vi "ActionVIOnLoad.vi"(8 "error in (no error)":errorcluster, 11 "Device Item Ref in":T1 format="%.0x") -> (0 "error out":errorcluster, 3 "Device Item Ref out":T1 format="%.0x")   [LabVIEW 2015, in "Diagnostics Addon System Explorer.lvlib"]
uses:
  Diagnostics Addon System Explorer.lvlib
  <vilib>/NI Veristand/Custom Device API/Custom Device Item Ref.ctl
  Shared/Types/Signal.ctl
  Shared/Types/986x.ctl
  Types/FG.Action.ctl
  Shared/Types/CAN.ctl
  Shared/Types/CAN.Interface.ctl
  Shared/Types/Protocol.ctl
  Shared/Types/Transport.ctl
  Shared/Types/Security.ctl
  Shared/Types/Type.ctl
  <vilib>/NI Veristand/Custom Device API/Custom Device Channel.ctl
  <vilib>/NI Veristand/Custom Device API/Custom Device Channel Type.ctl
  NationalInstruments.VeriStand.SystemDefinitionAPI
  SubVIs/FileDependency.Create.vi
  SubVIs/ID.FG.vi
  Shared/SubVIs/Constants.vi
  <vilib>/NI Veristand/Custom Device Tools/Custom Device Utility Library/NI VeriStand - Search for All Items by GUID.vi
  <vilib>/NI Veristand/Custom Device API/Get Item Property (Variant).vi
  <vilib>/NI Veristand/Custom Device API/Set Item Property (Variant).vi
  <vilib>/NI Veristand/Custom Device API/Get Item Property (U32).vi
  <vilib>/NI Veristand/Custom Device API/Get Item Property (Boolean).vi
  SubVIs/FileDependency.Get.Target Path.vi
  <vilib>/NI/NIVS System Definition Utilities/SysDef API/SysDef.Property.Set.vi
  <vilib>/NI/NIVS System Definition Utilities/_SubVIs/SysDef.Property.Set.U32.vi
  <vilib>/NI/NIVS System Definition Utilities/_SubVIs/SysDef.Property.Set.Boolean.vi
  <vilib>/Utility/MD5Checksum.llb/MD5Checksum File.vi
  <vilib>/NI/NIVS System Definition Utilities/_SubVIs/SysDef.Property.Set.DependentFile.vi
  <vilib>/NI/NIVS System Definition Utilities/SysDef API/SysDef.Property.Remove.vi
  <vilib>/NI Veristand/Custom Device API/Get Item Property (U16).vi
  <vilib>/NI Veristand/Custom Device API/Get Item Property (Path).vi
  <vilib>/NI Veristand/Custom Device Tools/Custom Device Utility Library/NI VeriStand - Search for Item by GUID.vi
  <vilib>/NI/NIVS System Definition Utilities/_SubVIs/SysDef.Property.Set.I32.vi
  <vilib>/NI Veristand/Custom Device API/Get Item Property (I32).vi
  <vilib>/NI/NIVS System Definition Utilities/_SubVIs/SysDef.Property.Set.U32.Array.vi
  <vilib>/NI Veristand/Custom Device API/Get Item Property (U32 Array).vi
  Shared/Diagnostics Addon Shared.lvlib
  <vilib>/NI VeriStand/Custom Device API/Custom Device API.lvlib
  <vilib>/NI Veristand/Custom Device Tools/Custom Device Utility Library/Custom Device Utility Library.lvlib
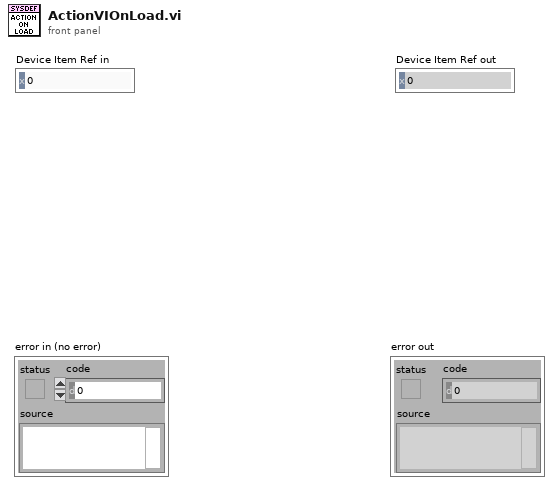
[diagram p1: front panel]
types:
  T1 = typedef "Custom Device API.lvlib/Custom Device Item Ref.ctl" = u64
  T2 = typedef "Diagnostics Addon Shared.lvlib/Signal.ctl" = cluster{"Start Bit":u32, "Length":u32, "Scaling Factor":dbl, "Scaling Offset":dbl, "Minimum":dbl, "Maximum":dbl, "Data Type":u32, "Byte Order":u32, "Default Value":dbl, "Name":string, "Units":string, "Description":string}
  T3 = cluster{"Name":string, "Start Bit":u8, "Length":u8, "Scaling Factor":dbl, "Scaling Offset":dbl, "Minimum":dbl, "Maximum":dbl, "Data Type":u32, "Byte Order":u32, "Default Value":dbl, "Units":string, "Description":string}
  T4 = cluster{"Start Bit":u8, "Length":u8, "Scaling Factor":dbl, "Scaling Offset":dbl, "Minimum":dbl, "Maximum":dbl, "Data Type":u32, "Byte Order":u32, "Default Value":dbl, "Name":string, "Units":string, "Description":string}
  T5 = typedef "Diagnostics Addon System Explorer.lvlib/FG.Action.ctl" = enum16{"Get", "Set"}
  T6 = typedef "Diagnostics Addon Shared.lvlib/986x.ctl" = cluster{"Enable":bool, "RIO Device":u16, "Bitfile":path}
  T7 = typedef "Custom Device API.lvlib/Custom Device Channel.ctl" = cluster{"Type":T8, "Units":string, "Default Value":dbl, "Faultable":bool, "Scalable":bool}
  T8 = typedef "Custom Device API.lvlib/Custom Device Channel Type.ctl" = enum16{"Input", "Output"}
  T9 = typedef "Diagnostics Addon Shared.lvlib/Type.ctl" = enum16{"DID", "CDID", "PID", "CPID", "Read Memory", "Write Memory", "DTC Control", "IO Cmd", "IO Resp", "Routine Start Cmd", "Routine Start Resp", "Routine Request Cmd", "Routine Request Resp", "Routine Stop Cmd", "Routine Stop Resp", "UserDefined Cmd", "UserDefined Rsp"}
  T10 = typedef "Diagnostics Addon Shared.lvlib/CAN.ctl" = cluster{"CAN Interface":T11, "Baud Rate":u32, "Diagnostic Protocol":T12, "Transport Protocol":T13, "Transmit ID":u32, "Receive ID":u32, "Transmit Extension":u8, "Receive Extension":u8, "Receive UUDT ID":u32, "Enable Stream":bool, "VW TP Channel ID":u32, "Security":T14, "Fill Frame":bool, "Fill Byte":u8, "Termination":bool}
  T11 = typedef "Diagnostics Addon Shared.lvlib/CAN.Interface.ctl" = enum16{"CAN0", "CAN1", "CAN2", "CAN3", "CAN4", "CAN5", "CAN6", "CAN7", "CAN8", "CAN9", "CAN10", "CAN11", "CAN12", "CAN13", "CAN14", "CAN15", "CAN16", "CAN17", "CAN18", "CAN19", "CAN20", "CAN21", "CAN22", "CAN23", "CAN24", "CAN25", "CAN26", "CAN27", "CAN28", "CAN29", "CAN30", "CAN31", "CAN32", "CAN33", "CAN34", "CAN35", "CAN36", "CAN37", "CAN38", "CAN39", "CAN40", "CAN41", "CAN42", "CAN43", "CAN44", "CAN45", "CAN46", "CAN47", "CAN48", "CAN49", "CAN50", "CAN51", "CAN52", "CAN53", "CAN54", "CAN55", "CAN56", "CAN57", "CAN58", "CAN59", "CAN60", "CAN61", "CAN62", "CAN63", "CAN 256 (Virtual)", "CAN 257 (Virtual)"}
  T12 = typedef "Diagnostics Addon Shared.lvlib/Protocol.ctl" = enum16{"GMLAN", "KWP-2000", "UDS", "User-Defined"}
  T13 = typedef "Diagnostics Addon Shared.lvlib/Transport.ctl" = enum16{"ISO TP - Normal Mode", "ISO TP - Mixed Mode", "VW TP 2.0", "Diagnostics on IP"}
  T14 = typedef "Diagnostics Addon Shared.lvlib/Security.ctl" = cluster{"Source DLL Path":path, "Security Level":u8, "Target DLL Path":path}
  T15 = cluster{"DTC Byte Length":i32, "Status Byte Length":i32, "Add Data Byte Length":i32, "Byte Order":enum16{"Motorola", "Intel"}}
  T16 = cluster{"Database File":path, "CAN Interface":enum16{"CAN0", "CAN1", "CAN2", "CAN3", "CAN4", "CAN5", "CAN6", "CAN7", "CAN8", "CAN9", "CAN10", "CAN11", "CAN12", "CAN13", "CAN14", "CAN15", "CAN16", "CAN17", "CAN18", "CAN19", "CAN20", "CAN21", "CAN22", "CAN23", "CAN24", "CAN25", "CAN26", "CAN27", "CAN28", "CAN29", "CAN30", "CAN31", "CAN32", "CAN33", "CAN34", "CAN35", "CAN36", "CAN37", "CAN38", "CAN39", "CAN40", "CAN41", "CAN42", "CAN43", "CAN44", "CAN45", "CAN46", "CAN47", "CAN48", "CAN49", "CAN50", "CAN51", "CAN52", "CAN53", "CAN54", "CAN55", "CAN56", "CAN57", "CAN58", "CAN59", "CAN60", "CAN61", "CAN62", "CAN63", "CAN 256 (Virtual)", "CAN 257 (Virtual)"}, "Baud Rate":u32, "Diagnostic Protocol":enum16{"GMLAN", "KWP-2000", "UDS"}, "Transport Protocol":enum16{"ISO TP - Normal Mode", "ISO TP - Mixed Mode", "VW TP 2.0", "Diagnostics on IP"}, "Transmit ID":u32, "Receive ID":u32, "Transmit Extension":u8, "Receive Extension":u8, "Receive UUDT ID":u32, "Enable Stream":bool, "VW TP Channel ID":u32}
  T17 = enum16{"CAN0", "CAN1", "CAN2", "CAN3", "CAN4", "CAN5", "CAN6", "CAN7", "CAN8", "CAN9", "CAN10", "CAN11", "CAN12", "CAN13", "CAN14", "CAN15", "CAN16", "CAN17", "CAN18", "CAN19", "CAN20", "CAN21", "CAN22", "CAN23", "CAN24", "CAN25", "CAN26", "CAN27", "CAN28", "CAN29", "CAN30", "CAN31", "CAN32", "CAN33", "CAN34", "CAN35", "CAN36", "CAN37", "CAN38", "CAN39", "CAN40", "CAN41", "CAN42", "CAN43", "CAN44", "CAN45", "CAN46", "CAN47", "CAN48", "CAN49", "CAN50", "CAN51", "CAN52", "CAN53", "CAN54", "CAN55", "CAN56", "CAN57", "CAN58", "CAN59", "CAN60", "CAN61", "CAN62", "CAN63", "CAN 256 (Virtual)", "CAN 257 (Virtual)"}
  T18 = enum16{"ISO TP - Normal Mode", "ISO TP - Mixed Mode", "VW TP 2.0", "Diagnostics on IP"}
  T19 = cluster{"DPID ID":u8, "Speed":enum16{"Slow", "Medium", "Fast"}, "PIDs":u16[]}
  T20 = typedef "Custom Device API.lvlib/Custom Device Item Info.ctl" = cluster{"Name":string, "Is Channel":bool, "GUID":string, "Is Waveform":bool}
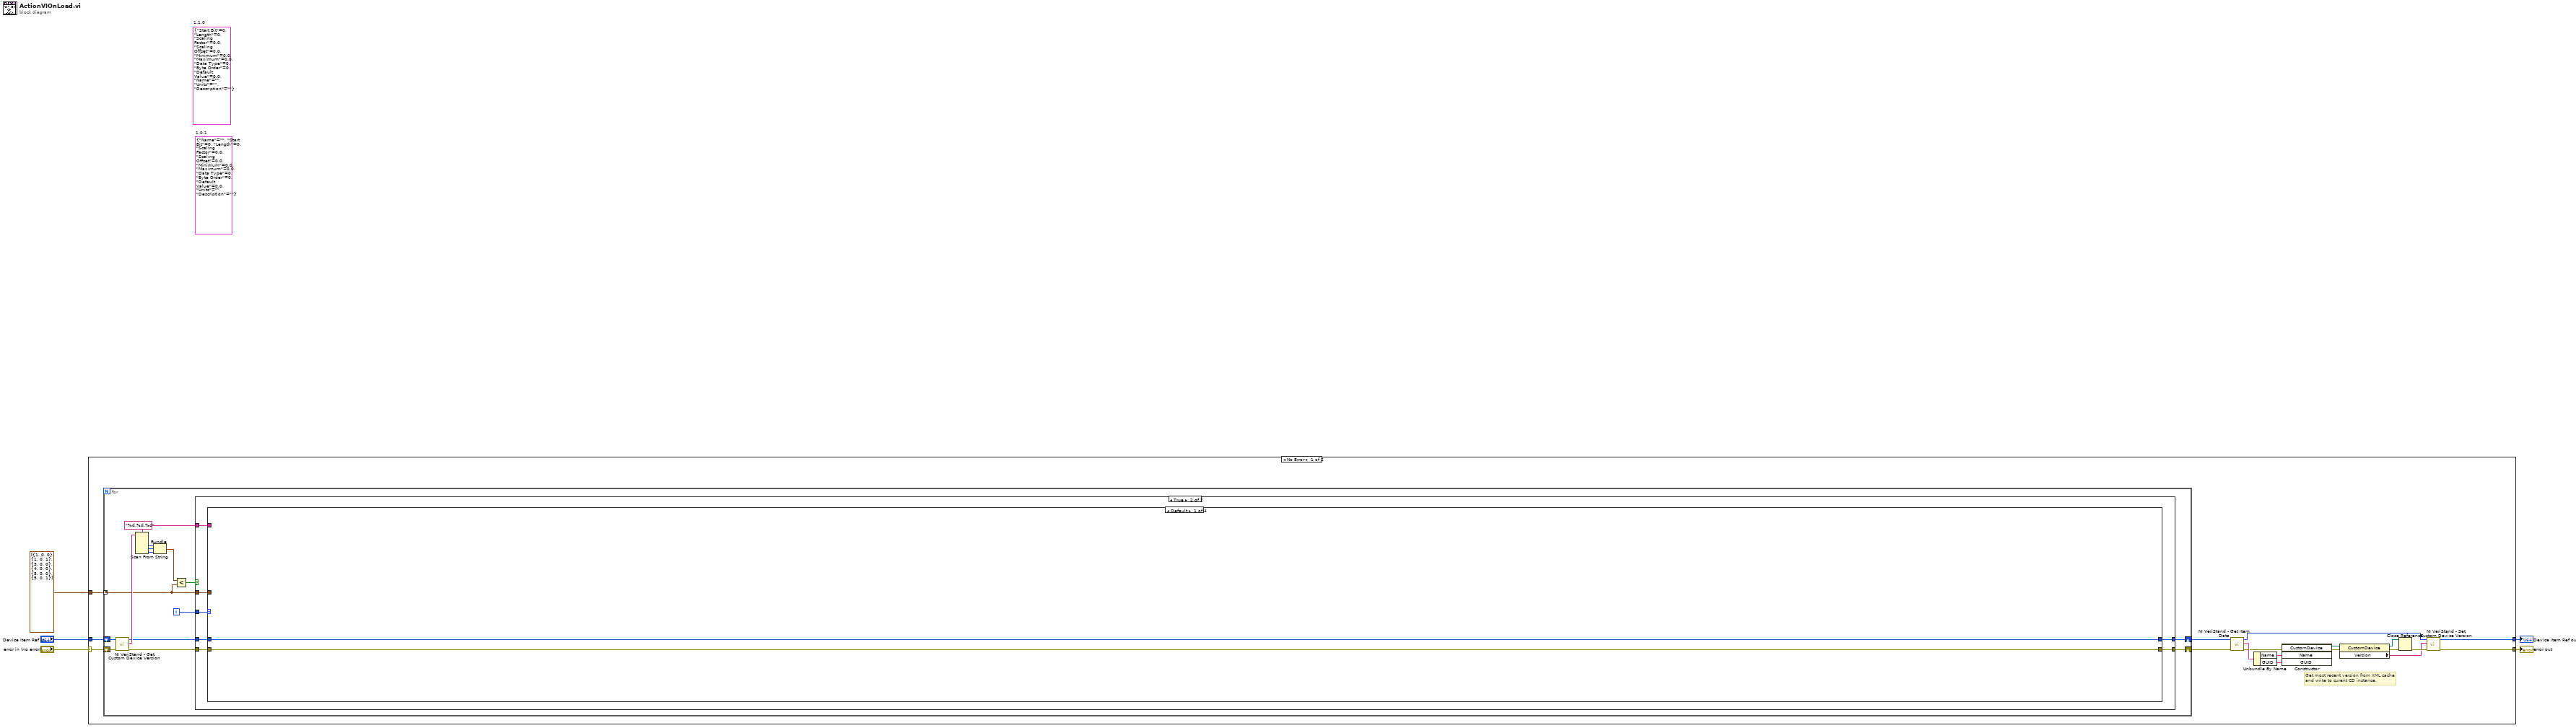
[diagram p0: block diagram]
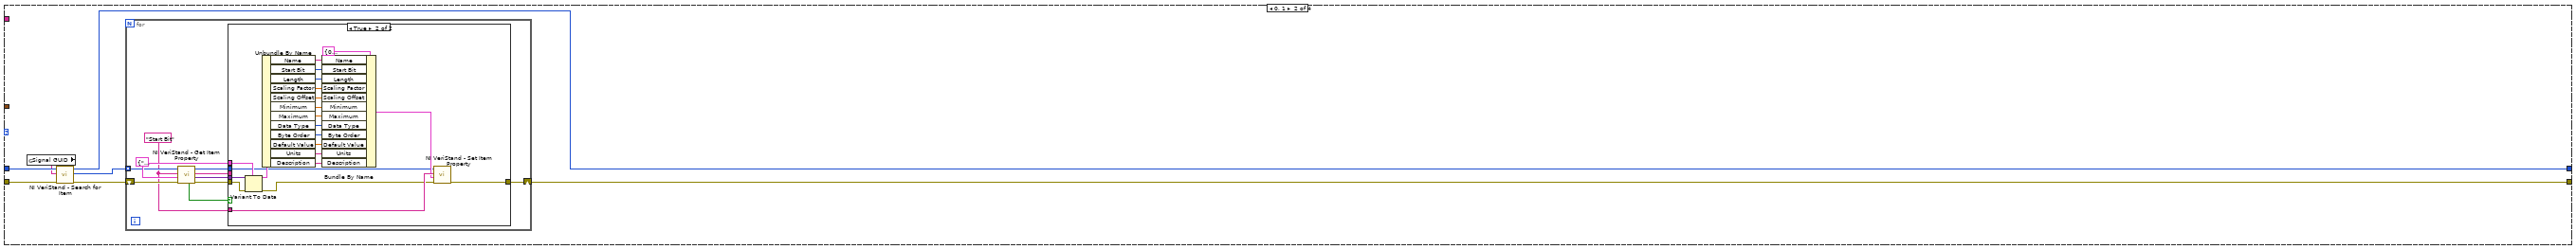
[diagram p3: hidden frame]
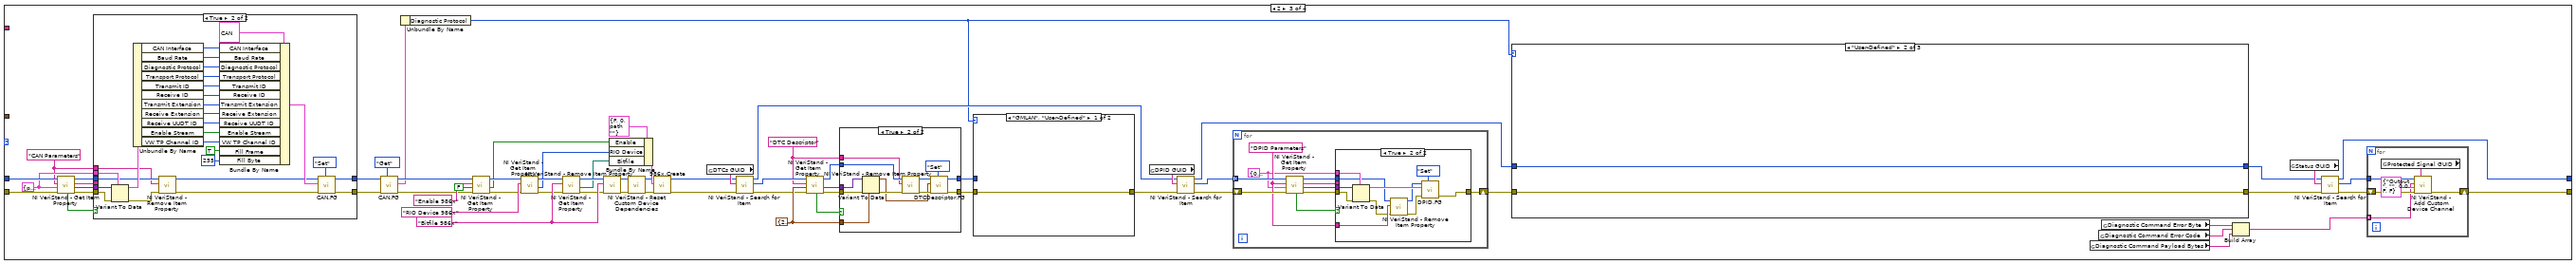
[diagram p5: hidden frame]
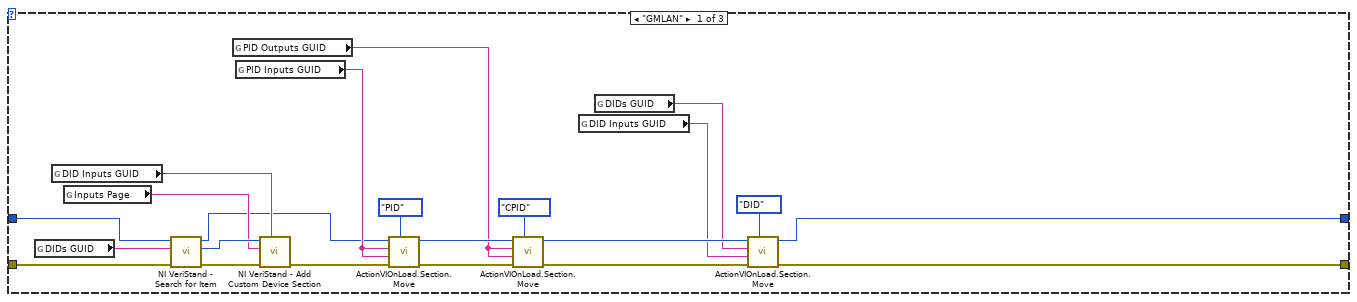
[diagram p6: hidden frame]
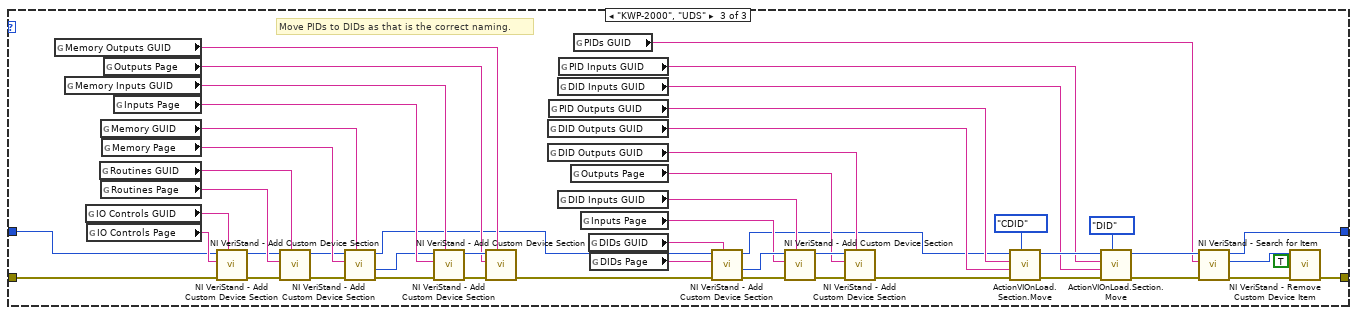
[diagram p7: hidden frame]
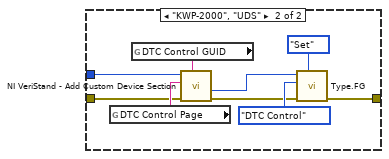
[diagram p8: hidden frame]
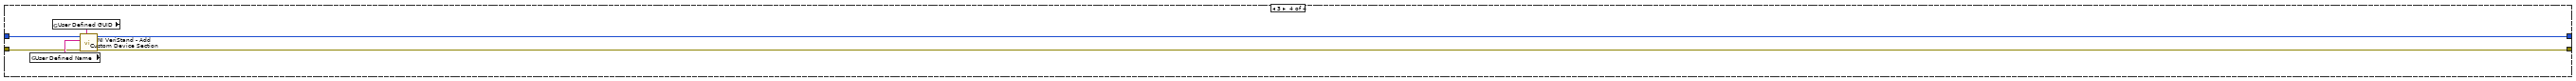
[diagram p12: hidden frame]
diagram:
  (unwired) T2 {"Start Bit"=0, "Length"=0, "Scaling Factor"=0.0, "Scaling Offset"=0.0, "Minimum"=0.0, "Maximum"=0.0, "Data Type"=0, "Byte Order"=0, "Default Value"=0.0, "Name"="", "Units"="", "Description"=""}  # 1.1.0
  (unwired) T3 {"Name"="", "Start Bit"=0, "Length"=0, "Scaling Factor"=0.0, "Scaling Offset"=0.0, "Minimum"=0.0, "Maximum"=0.0, "Data Type"=0, "Byte Order"=0, "Default Value"=0.0, "Units"="", "Description"=""}  # 1.0.1
  n1 = case shown="No Error" "error in (no error)" {
    selector: "error in (no error)" -> [w22 w315]
    tunnel: [w8 w315] -> w2
    tunnel: "Device Item Ref in" -> [w21 w314]
    tunnel: [w6 w314] -> w1
    tunnel: cluster{i32, i32, i32}[] [{1, 0, 0}, {1, 0, 1}, {3, 0, 0}, {4, 0, 0}, {5, 0, 0}, {5, 0, 1}] -> [w23 _]
    frame No Error {
      # "Get most recent version from XML cache\nand write to curent CD instance."
      n2 = for {
        tunnel: w23 -> [w26] mode=indexing
        shift-right: [w31] -> w9
        shift-left: w22 -> [w36]
        shift-right: [w29] -> w7
        shift-left: w21 -> [w35]
        i -> [w28]
        w27 = "%d.%d.%d" ("format string")
        n3 = call <vilib>:"NI VeriStand - Get Custom Device Version.vi"("error in (no error)"=w36, "Device Ref in"=w35) -> ("error out"=w32:errorcluster, "Value"=w34:string, "Device Ref out"=w30:T1)  [unwired: 7 in]
        n4 = Scan From String(format string=w27, input string=w34) -> (output 1=w37:i32, output 2=w38:i32, output 3=w25:i32)  [unwired: 5 in, 3 out]
        n5 = Bundle(w37, w38, w25) -> (w24:cluster{i32, i32, i32})  [unwired: 1 in]
        n6 = Less?(x=w24, y=w26) -> (x < y?=w33:bool)
        n7 = case shown="True" w33 {
          tunnel: w32 -> [w40 w47]
          tunnel: [w40 w46] -> w31
          tunnel: w30 -> [w39 w43]
          tunnel: [w39 w44] -> w29
          tunnel: w28 -> [_ w45]
          tunnel: w26 -> [_ w42]
          tunnel: w27 -> [_ w41]
          frame False {
          }
          frame True {
            n8 = case shown="Default" w45 {
              tunnel: w47 -> [w49 w55 w149 w311]
              tunnel: [w49 w51 w90 w309] -> w46
              tunnel: [w48 w50 w89 w308] -> w44
              tunnel: w43 -> [w48 w56 w148 w310]
              tunnel: w42 -> [_ _ _ _]
              tunnel: w41 -> [_ _ _ _]
              frame Default {
              }
              frame 0, 1 {
                n9 = global read "Constants.vi" "Signal GUID"() -> (w54:string)
                n10 = call-poly <vilib>:"NI VeriStand - Search for Item.vi"("error in"=w55, "Item GUID"=w54, "Section Ref in"=w56) -> ("error out"=w53:errorcluster, "Item Refs"=w52:T1[], "Section Ref out"=w50:T1)  [unwired: 5 in, 1 out]
                n11 = for {
                  shift-right: [w60] -> w51
                  shift-left: w53 -> [w61]
                  tunnel: w52 -> [w58] mode=indexing
                  w57 = "Start Bit" ("DIDPID Signal Parameters")
                  w62 = T3 {"Name"="", "Start Bit"=0, "Length"=0, "Scaling Factor"=0.0, "Scaling Offset"=0.0, "Minimum"=0.0, "Maximum"=0.0, "Data Type"=0, "Byte Order"=0, "Default Value"=0.0, "Units"="", "Description"=""} ("Signal Parameters")
                  n12 = call-poly <vilib>:"NI VeriStand - Get Item Property.vi"("error in (no error)"=w61, "Default Value"=w62, "Property Name"=w57, "Item Ref in"=w58) -> ("error out"=w64:errorcluster, "Value"=w63:variant, "Item Ref out"=w59:T1, "Found?"=w65:bool)  [unwired: 4 in]
                  n13 = case shown="True" w65 {
                    tunnel: w64 -> [w66 w88]
                    tunnel: w63 -> [_ w87]
                    tunnel: w62 -> [_ w86]
                    tunnel: [w66 w67] -> w60
                    tunnel: w59 -> [_ w69]
                    tunnel: w57 -> [_ _]
                    tunnel: w57 -> [_ w71]
                    frame False {
                    }
                    frame True {
                      n14 = Variant To Data(error in=w88, type=w86, Variant=w87) -> (data=w85:T3, error out=w68:errorcluster)
                      n15 = Unbundle By Name(w85) -> ("Name"=w84:string, "Start Bit"=w83:u8, "Length"=w82:u8, "Scaling Factor"=w81:dbl, "Scaling Offset"=w80:dbl, "Minimum"=w79:dbl, "Maximum"=w78:dbl, "Data Type"=w77:u32, "Byte Order"=w76:u32, "Default Value"=w75:dbl, "Units"=w74:string, "Description"=w73:string)
                      n16 = Bundle By Name(cluster=T4 {"Start Bit"=0, "Length"=0, "Scaling Factor"=0.0, "Scaling Offset"=0.0, "Minimum"=0.0, "Maximum"=0.0, "Data Type"=0, "Byte Order"=0, "Default Value"=0.0, "Name"="", "Units"="", "Description"=""} ("Signal Parameters"), "Name"=w84, "Start Bit"=w83, "Length"=w82, "Scaling Factor"=w81, "Scaling Offset"=w80, "Minimum"=w79, "Maximum"=w78, "Data Type"=w77, "Byte Order"=w76, "Default Value"=w75, "Units"=w74, "Description"=w73) -> (w70:T4)
                      n17 = call-poly <vilib>:"NI VeriStand - Set Item Property.vi"("error in (no error)"=w68, "Value"=w70, "Property Name"=w71, "Item Ref in"=w69) -> ("error out"=w67:errorcluster)  [unwired: 5 in, 2 out]
                    }
                  }
                }
              }
              frame 2 {
                w129 = T15 {"DTC Byte Length"=2, "Status Byte Length"=1, "Add Data Byte Length"=1, "Byte Order"=enum."Motorola"} ("DTC descriptor")
                w122 = "DTC Descriptor" ("DTC Descriptor")
                w143 = "Bitfile 986x" ("Bitfile 986x")
                w106 = "CAN Parameters" ("DIDPID Signal Parameters")
                w147 = T16 {"Database File"=path "", "CAN Interface"=enum."CAN0", "Baud Rate"=0, "Diagnostic Protocol"=enum."GMLAN", "Transport Protocol"=enum."ISO TP - Normal Mode", "Transmit ID"=0, "Receive ID"=0, "Transmit Extension"=0, "Receive Extension"=0, "Receive UUDT ID"=0, "Enable Stream"=TRUE, "VW TP Channel ID"=0} ("Diagnostics Basic Configuraiton")
                n18 = call-poly <vilib>:"NI VeriStand - Get Item Property.vi"("error in (no error)"=w149, "Default Value"=w147, "Property Name"=w106, "Item Ref in"=w148) -> ("error out"=w152:errorcluster, "Value"=w151:variant, "Item Ref out"=w150:T1, "Found?"=w153:bool)  [unwired: 4 in]
                n19 = case shown="True" w153 {
                  tunnel: w152 -> [w280 w307]
                  tunnel: w151 -> [_ w306]
                  tunnel: w147 -> [_ w305]
                  tunnel: [w280 w290] -> w112
                  tunnel: w150 -> [w279 w283]
                  tunnel: w106 -> [_ _]
                  tunnel: [w279 w288] -> w110
                  tunnel: w106 -> [_ w281]
                  frame False {
                  }
                  frame True {
                    n20 = Variant To Data(error in=w307, type=w305, Variant=w306) -> (data=w304:T16, error out=w285:errorcluster)
                    n21 = Unbundle By Name(w304) -> ("CAN Interface"=w303:T17, "Baud Rate"=w302:u32, "Diagnostic Protocol"=w301:enum16{"GMLAN", "KWP-2000", "UDS"}, "Transport Protocol"=w300:T18, "Transmit ID"=w299:u32, "Receive ID"=w298:u32, "Transmit Extension"=w297:u8, "Receive Extension"=w296:u8, "Receive UUDT ID"=w295:u32, "Enable Stream"=w294:bool, "VW TP Channel ID"=w293:u32)
                    n22 = call <vilib>:"NI VeriStand - Remove Item Property.vi"("error in (no error)"=w285, "Property Name"=w281, "Item Ref in"=w283) -> ("error out"=w284:errorcluster, "Item Ref out"=w282:T1)  [unwired: 6 in, 1 out]
                    n23 = Bundle By Name(cluster=T10 {"CAN Interface"=enum."CAN0", "Baud Rate"=0, "Diagnostic Protocol"=enum."GMLAN", "Transport Protocol"=enum."ISO TP - Normal Mode", "Transmit ID"=0, "Receive ID"=0, "Transmit Extension"=0, "Receive Extension"=0, "Receive UUDT ID"=0, "Enable Stream"=TRUE, "VW TP Channel ID"=0, "Security"={"Source DLL Path"=path "", "Security Level"=1, "Target DLL Path"=path ""}, "Fill Frame"=FALSE, "Fill Byte"=255, "Termination"=FALSE} ("Diagnostics Basic Configuraiton"), "CAN Interface"=w303, "Baud Rate"=w302, "Diagnostic Protocol"=w301, "Transport Protocol"=w300, "Transmit ID"=w299, "Receive ID"=w298, "Transmit Extension"=w297, "Receive Extension"=w296, "Receive UUDT ID"=w295, "Enable Stream"=w294, "VW TP Channel ID"=w293, "Fill Frame"=TRUE, "Fill Byte"=u8 255) -> (w289:T10)
                    n24 = call "CAN.FG.vi"("Action"=FG.Action."Set", "error in (no error)"=w284, "Diagnostics Basic Configuraiton"=w289, "Device Item Ref in"=w282) -> ("error out"=w290:errorcluster, "Device Item Ref out"=w288:T1)  [unwired: 5 in, 1 out]
                  }
                }
                n25 = call "CAN.FG.vi"("Action"=FG.Action."Get", "error in (no error)"=w112, "Device Item Ref in"=w110) -> ("error out"=w111:errorcluster, "Diagnostics Basic Configuraiton"=w108:T10, "Device Item Ref out"=w109:T1)  [unwired: 6 in]
                n26 = Unbundle By Name(w108) -> ("Diagnostic Protocol"=w91:T12)
                n27 = call-poly <vilib>:"NI VeriStand - Get Item Property.vi"("error in (no error)"=w111, "Default Value"=FALSE, "Property Name"="Enable 986x" ("Enable 986x"), "Item Ref in"=w109) -> ("error out"=w140:errorcluster, "Value"=w136:bool, "Item Ref out"=w139:T1)  [unwired: 4 in, 1 out]
                n28 = call-poly <vilib>:"NI VeriStand - Get Item Property.vi"("error in (no error)"=w140, "Property Name"="RIO Device 986x" ("RIO Device 986x"), "Item Ref in"=w139) -> ("error out"=w141:errorcluster, "Value"=w135:u16, "Item Ref out"=w138:T1)  [unwired: 5 in, 1 out]
                n29 = call-poly <vilib>:"NI VeriStand - Get Item Property.vi"("error in (no error)"=w141, "Property Name"=w143, "Item Ref in"=w138) -> ("error out"=w142:errorcluster, "Value"=w134:path, "Item Ref out"=w144:T1)  [unwired: 5 in, 1 out]
                n30 = call <vilib>:"NI VeriStand - Remove Item Property.vi"("error in (no error)"=w142, "Property Name"=w143, "Item Ref in"=w144) -> ("error out"=w102:errorcluster, "Item Ref out"=w132:T1)  [unwired: 6 in, 1 out]
                n31 = Bundle By Name(cluster=T6 {"Enable"=FALSE, "RIO Device"=0, "Bitfile"=path ""} ("986x Support"), "Enable"=w136, "RIO Device"=w135, "Bitfile"=w134) -> (w133:T6)
                n32 = call <vilib>:"NI VeriStand - Reset Custom Device Dependencies.vi"("error in (no error)"=w102, "Device Ref in"=w132) -> ("error out"=w101:errorcluster, "Device Ref out"=w103:T1)  [unwired: 8 in]
                n33 = call "986x.Create.vi"("error in (no error)"=w101, "986x Support"=w133, "Device Item Ref in"=w103) -> ("error out"=w105:errorcluster, "Device Ref out"=w104:T1)  [unwired: 7 in]
                n34 = global read "Constants.vi" "DTCs GUID"() -> (w130:string)
                n35 = call-poly <vilib>:"NI VeriStand - Search for Item.vi"("error in"=w105, "Item GUID"=w130, "Section Ref in"=w104) -> ("error out"=w125:errorcluster, "Item Ref"=w124:T1, "Section Ref out"=w115:T1)  [unwired: 5 in, 1 out]
                n36 = call-poly <vilib>:"NI VeriStand - Get Item Property.vi"("error in (no error)"=w125, "Default Value"=w129, "Property Name"=w122, "Item Ref in"=w124) -> ("error out"=w128:errorcluster, "Value"=w127:variant, "Item Ref out"=w123:T1, "Found?"=w126:bool)  [unwired: 4 in]
                n37 = case shown="True" w126 {
                  tunnel: w128 -> [w266 w278]
                  tunnel: [w266 w269] -> w118
                  tunnel: w127 -> [_ w277]
                  tunnel: w129 -> [_ w276]
                  tunnel: w123 -> [w265 w274]
                  tunnel: w122 -> [_ w268]
                  tunnel: [w265 w267] -> w117
                  frame False {
                  }
                  frame True {
                    n38 = Variant To Data(error in=w278, type=w276, Variant=w277) -> (data=w270:T15, error out=w275:errorcluster)
                    n39 = call <vilib>:"NI VeriStand - Remove Item Property.vi"("error in (no error)"=w275, "Property Name"=w268, "Item Ref in"=w274) -> ("error out"=w271:errorcluster, "Item Ref out"=w272:T1)  [unwired: 6 in, 1 out]
                    n40 = call "DTCDescriptor.FG.vi"("Action"=FG.Action."Set", "error in (no error)"=w271, "DTC descriptor"=w270, "Device Item Ref in"=w272) -> ("error out"=w269:errorcluster, "Device Item Ref out"=w267:T1)  [unwired: 5 in, 1 out]
                  }
                }
                n41 = case shown="\"GMLAN\", \"User-Defined\"" w91 {
                  tunnel: w118 -> [w234 w238]
                  tunnel: w117 -> [_ w237]
                  tunnel: [w234 w236] -> w116
                  frame "GMLAN", "User-Defined" {
                  }
                  frame "KWP-2000", "UDS" {
                    n42 = global read "Constants.vi" "DTC Control Page"() -> (w243:string)
                    n43 = global read "Constants.vi" "DTC Control GUID"() -> (w242:string)
                    n44 = call <vilib>:"NI VeriStand - Add Custom Device Section.vi"("GUID (Default Section)"=w242, "error in (no error)"=w238, "Section Name"=w243, "Parent Ref in"=w237) -> ("error out"=w239:errorcluster, "Section Ptr"=w235:T1)  [unwired: 4 in, 2 out]
                    n45 = call "Type.FG.vi"("Action"=FG.Action."Set", "error in (no error)"=w239, "Type"=Type."DTC Control", "Device Item Ref in"=w235) -> ("error out"=w236:errorcluster)  [unwired: 5 in, 2 out]
                  }
                }
                n46 = global read "Constants.vi" "DPID GUID"() -> (w120:string)
                n47 = call-poly <vilib>:"NI VeriStand - Search for Item.vi"("error in"=w116, "Item GUID"=w120, "Section Ref in"=w115) -> ("error out"=w119:errorcluster, "Item Refs"=w121:T1[], "Section Ref out"=w107:T1)  [unwired: 5 in, 1 out]
                n48 = for {
                  shift-right: [w248] -> w114
                  shift-left: w119 -> [w249]
                  tunnel: w121 -> [w246] mode=indexing
                  w244 = T19 {"DPID ID"=0, "Speed"=enum."Slow", "PIDs"=[]} ("DPID")
                  w245 = "DPID Parameters" ("DPID Parameters")
                  n49 = call-poly <vilib>:"NI VeriStand - Get Item Property.vi"("error in (no error)"=w249, "Default Value"=w244, "Property Name"=w245, "Item Ref in"=w246) -> ("error out"=w251:errorcluster, "Value"=w250:variant, "Item Ref out"=w247:T1, "Found?"=w252:bool)  [unwired: 4 in]
                  n50 = case shown="True" w252 {
                    tunnel: w251 -> [w253 w264]
                    tunnel: w250 -> [_ w263]
                    tunnel: w244 -> [_ w262]
                    tunnel: [w253 w256] -> w248
                    tunnel: w247 -> [_ w255]
                    tunnel: w245 -> [_ _]
                    tunnel: w245 -> [_ w261]
                    frame False {
                    }
                    frame True {
                      n51 = Variant To Data(error in=w264, type=w262, Variant=w263) -> (data=w260:T19, error out=w258:errorcluster)
                      n52 = call <vilib>:"NI VeriStand - Remove Item Property.vi"("error in (no error)"=w258, "Property Name"=w261, "Item Ref in"=w255) -> ("error out"=w257:errorcluster, "Item Ref out"=w254:T1)  [unwired: 6 in, 1 out]
                      n53 = call "DPID.FG.vi"("Action"=FG.Action."Set", "error in (no error)"=w257, "DPID"=w260, "Device Item Ref in"=w254) -> ("error out"=w256:errorcluster)  [unwired: 5 in, 2 out]
                    }
                  }
                }
                n54 = case shown="\"User-Defined\"" w91 {
                  tunnel: [w168 w182 w189] -> w92
                  tunnel: [w164 w183 w185] -> w94
                  tunnel: w114 -> [w166 w183 w215]
                  tunnel: w107 -> [w180 w182 w214]
                  frame "GMLAN" {
                    n55 = global read "Constants.vi" "DIDs GUID"() -> (w181:string)
                    n56 = global read "Constants.vi" "DID Inputs GUID"() -> (w177:string)
                    n57 = global read "Constants.vi" "Inputs Page"() -> (w176:string)
                    n58 = call-poly <vilib>:"NI VeriStand - Search for Item.vi"("error in"=w166, "Item GUID"=w181, "Section Ref in"=w180) -> ("error out"=w179:errorcluster, "Item Ref"=w178:T1, "Section Ref out"=w163:T1)  [unwired: 5 in, 1 out]
                    n59 = global read "Constants.vi" "PID Outputs GUID"() -> (w170:string)
                    n60 = global read "Constants.vi" "PID Inputs GUID"() -> (w171:string)
                    n61 = call <vilib>:"NI VeriStand - Add Custom Device Section.vi"("GUID (Default Section)"=w177, "error in (no error)"=w179, "Section Name"=w176, "Parent Ref in"=w178) -> ("error out"=w165:errorcluster)  [unwired: 4 in, 3 out]
                    n62 = call "ActionVIOnLoad.Section.Move.vi"("Type"=Type."PID", "error in (no error)"=w165, "Paste Parent GUID"=w171, "Copy Parent GUID"=w171, "Section Ref in"=w163) -> ("error out"=w175:errorcluster, "Section Ref out"=w174:T1)  [unwired: 5 in]
                    n63 = call "ActionVIOnLoad.Section.Move.vi"("Type"=Type."CPID", "error in (no error)"=w175, "Paste Parent GUID"=w170, "Copy Parent GUID"=w170, "Section Ref in"=w174) -> ("error out"=w167:errorcluster, "Section Ref out"=w169:T1)  [unwired: 5 in]
                    n64 = global read "Constants.vi" "DID Inputs GUID"() -> (w161:string)
                    n65 = global read "Constants.vi" "DIDs GUID"() -> (w160:string)
                    n66 = call "ActionVIOnLoad.Section.Move.vi"("Type"=Type."DID", "error in (no error)"=w167, "Paste Parent GUID"=w161, "Copy Parent GUID"=w160, "Section Ref in"=w169) -> ("error out"=w164:errorcluster, "Section Ref out"=w168:T1)  [unwired: 5 in]
                  }
                  frame "User-Defined" {
                  }
                  frame "KWP-2000", "UDS" {
                    # "Move PIDs to DIDs as that is the correct naming."
                    n67 = global read "Constants.vi" "Memory Outputs GUID"() -> (w221:string)
                    n68 = global read "Constants.vi" "Memory Inputs GUID"() -> (w225:string)
                    n69 = global read "Constants.vi" "IO Controls GUID"() -> (w231:string)
                    n70 = global read "Constants.vi" "IO Controls Page"() -> (w230:string)
                    n71 = global read "Constants.vi" "Routines GUID"() -> (w232:string)
                    n72 = global read "Constants.vi" "Memory GUID"() -> (w228:string)
                    n73 = global read "Constants.vi" "Routines Page"() -> (w233:string)
                    n74 = global read "Constants.vi" "Memory Page"() -> (w227:string)
                    n75 = global read "Constants.vi" "Outputs Page"() -> (w222:string)
                    n76 = global read "Constants.vi" "Inputs Page"() -> (w224:string)
                    n77 = call <vilib>:"NI VeriStand - Add Custom Device Section.vi"("GUID (Default Section)"=w231, "error in (no error)"=w215, "Section Name"=w230, "Parent Ref in"=w214) -> ("error out"=w217:errorcluster, "Parent Ref out"=w229:T1)  [unwired: 4 in, 2 out]
                    n78 = call <vilib>:"NI VeriStand - Add Custom Device Section.vi"("GUID (Default Section)"=w232, "error in (no error)"=w217, "Section Name"=w233, "Parent Ref in"=w229) -> ("error out"=w216:errorcluster, "Parent Ref out"=w226:T1)  [unwired: 4 in, 2 out]
                    n79 = call <vilib>:"NI VeriStand - Add Custom Device Section.vi"("GUID (Default Section)"=w228, "error in (no error)"=w216, "Section Name"=w227, "Parent Ref in"=w226) -> ("error out"=w220:errorcluster, "Section Ptr"=w219:T1, "Parent Ref out"=w203:T1)  [unwired: 4 in, 1 out]
                    n80 = call <vilib>:"NI VeriStand - Add Custom Device Section.vi"("GUID (Default Section)"=w225, "error in (no error)"=w220, "Section Name"=w224, "Parent Ref in"=w219) -> ("error out"=w218:errorcluster, "Parent Ref out"=w223:T1)  [unwired: 4 in, 2 out]
                    n81 = call <vilib>:"NI VeriStand - Add Custom Device Section.vi"("GUID (Default Section)"=w221, "error in (no error)"=w218, "Section Name"=w222, "Parent Ref in"=w223) -> ("error out"=w209:errorcluster)  [unwired: 4 in, 3 out]
                    n82 = global read "Constants.vi" "DID Outputs GUID"() -> (w198:string)
                    n83 = global read "Constants.vi" "DID Outputs GUID"() -> (w205:string)
                    n84 = global read "Constants.vi" "PID Outputs GUID"() -> (w200:string)
                    n85 = global read "Constants.vi" "DID Inputs GUID"() -> (w193:string)
                    n86 = global read "Constants.vi" "DID Inputs GUID"() -> (w211:string)
                    n87 = global read "Constants.vi" "PID Inputs GUID"() -> (w192:string)
                    n88 = global read "Constants.vi" "Outputs Page"() -> (w206:string)
                    n89 = global read "Constants.vi" "PIDs GUID"() -> (w188:string)
                    n90 = global read "Constants.vi" "Inputs Page"() -> (w210:string)
                    n91 = global read "Constants.vi" "DIDs GUID"() -> (w208:string)
                    n92 = global read "Constants.vi" "DIDs Page"() -> (w202:string)
                    n93 = call <vilib>:"NI VeriStand - Add Custom Device Section.vi"("GUID (Default Section)"=w208, "error in (no error)"=w209, "Section Name"=w202, "Parent Ref in"=w203) -> ("error out"=w213:errorcluster, "Section Ptr"=w212:T1, "Parent Ref out"=w197:T1)  [unwired: 4 in, 1 out]
                    n94 = call <vilib>:"NI VeriStand - Add Custom Device Section.vi"("GUID (Default Section)"=w211, "error in (no error)"=w213, "Section Name"=w210, "Parent Ref in"=w212) -> ("error out"=w204:errorcluster, "Parent Ref out"=w207:T1)  [unwired: 4 in, 2 out]
                    n95 = call <vilib>:"NI VeriStand - Add Custom Device Section.vi"("GUID (Default Section)"=w205, "error in (no error)"=w204, "Section Name"=w206, "Parent Ref in"=w207) -> ("error out"=w201:errorcluster)  [unwired: 4 in, 3 out]
                    n96 = call "ActionVIOnLoad.Section.Move.vi"("Type"=Type."CDID", "error in (no error)"=w201, "Paste Parent GUID"=w198, "Copy Parent GUID"=w200, "Section Ref in"=w197) -> ("error out"=w196:errorcluster, "Section Ref out"=w195:T1)  [unwired: 5 in]
                    n97 = call "ActionVIOnLoad.Section.Move.vi"("Type"=Type."DID", "error in (no error)"=w196, "Paste Parent GUID"=w193, "Copy Parent GUID"=w192, "Section Ref in"=w195) -> ("error out"=w191:errorcluster, "Section Ref out"=w190:T1)  [unwired: 5 in]
                    n98 = call-poly <vilib>:"NI VeriStand - Search for Item.vi"("error in"=w191, "Item GUID"=w188, "Section Ref in"=w190) -> ("error out"=w186:errorcluster, "Item Ref"=w184:T1, "Section Ref out"=w189:T1)  [unwired: 5 in, 1 out]
                    n99 = call <vilib>:"NI VeriStand - Remove Custom Device Item.vi"("error in (no error)"=w186, "Force Delete (F)"=TRUE, "Item Ref in"=w184) -> ("error out"=w185:errorcluster)  [unwired: 7 in, 1 out]
                  }
                }
                n100 = global read "Constants.vi" "Diagnostic Command Payload Bytes"() -> (w99:string)
                n101 = global read "Constants.vi" "Diagnostic Command Error Code"() -> (w98:string)
                n102 = global read "Constants.vi" "Diagnostic Command Error Byte"() -> (w100:string)
                n103 = Build Array(w100, w98, w99) -> (w97:string[])
                n104 = global read "Constants.vi" "Status GUID"() -> (w96:string)
                n105 = call-poly <vilib>:"NI VeriStand - Search for Item.vi"("error in"=w94, "Item GUID"=w96, "Section Ref in"=w92) -> ("error out"=w93:errorcluster, "Item Ref"=w95:T1, "Section Ref out"=w89:T1)  [unwired: 5 in, 1 out]
                n106 = for {
                  tunnel: w95 -> [w157]
                  shift-right: [w156] -> w90
                  shift-left: w93 -> [w158]
                  tunnel: w97 -> [w155] mode=indexing
                  n107 = global read "Constants.vi" "Protected Signal GUID"() -> (w154:string)
                  n108 = call <vilib>:"NI VeriStand - Add Custom Device Channel.vi"("GUID (Default Channel)"=w154, "error in (no error)"=w158, "Channel"=T7 {"Type"=enum."Output", "Units"="", "Default Value"=0.0, "Faultable"=FALSE, "Scalable"=FALSE}, "Channel Name"=w155, "Parent Ref in"=w157) -> ("error out"=w156:errorcluster)  [unwired: 3 in, 3 out]
                }
              }
              frame 3 {
                n109 = global read "Constants.vi" "User Defined Name"() -> (w312:string)
                n110 = global read "Constants.vi" "User Defined GUID"() -> (w313:string)
                n111 = call <vilib>:"NI VeriStand - Add Custom Device Section.vi"("GUID (Default Section)"=w313, "error in (no error)"=w311, "Section Name"=w312, "Parent Ref in"=w310) -> ("error out"=w309:errorcluster, "Parent Ref out"=w308:T1)  [unwired: 4 in, 2 out]
              }
            }
          }
        }
      }
      n112 = call <vilib>:"NI VeriStand - Get Item Data.vi"("error in (no error)"=w9, "Item Ref in"=w7) -> ("error out"=w17:errorcluster, "Item Info"=w20:T20, "Item Ref out"=w10:T1)  [unwired: 6 in, 1 out]
      n113 = Unbundle By Name(w20) -> ("Name"=w19:string, "GUID"=w18:string)
      n114 = constructor class="CustomDevice"(error in=w17, "Name"=w19, "GUID"=w18) -> (reference out=w16:refnum<k24>, error out=w15:errorcluster)  [unwired: 2 in, 3 out]
      n115 = property class="CustomDevice"(reference=w16, error in=w15) -> (reference out=w13:refnum<k24>, error out=w14:errorcluster, "Version"=w11:string)
      n116 = Close Reference(reference=w13, error in (no error)=w14) -> (error out=w12:errorcluster)
      n117 = call <vilib>:"NI VeriStand - Set Custom Device Version.vi"("error in (no error)"=w12, "Value"=w11, "Device Ref in"=w10) -> ("error out"=w8:errorcluster, "Device Ref out"=w6:T1)  [unwired: 7 in]
    }
    frame Error {
    }
  }
  "error out" <- w2
  "Device Item Ref out" <- w1
